vi "CRYGet Group Category.vi"(7 "sOption":string, 11 "nData":i32) -> (3 "sCategory":string)   [LabVIEW 2013]
uses:
  CRYProject/CRYProject Editor Global.vi
  Global/CRYCurve Library Global.vi
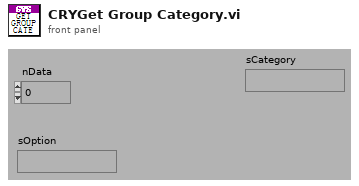
[diagram p1: front panel]
types:
  T1 = typedef "CRYStep.ctl" = cluster{"No.VI":i32, "Category":string, "StepName":string, "Seq setup flattened":string, "Comment":string, "Steps config.":bool[], "Jump config":i32[], "Start":dbl, "Increment":dbl, "Name":string, "Unit":string, "Y data":u16, "Y prefix":string, "Y dB ref":dbl, "Y unit":string, "Repeat State Array":cluster{"Start":dbl, "Increment":dbl, "Count":i32, "Num":i32}[]}
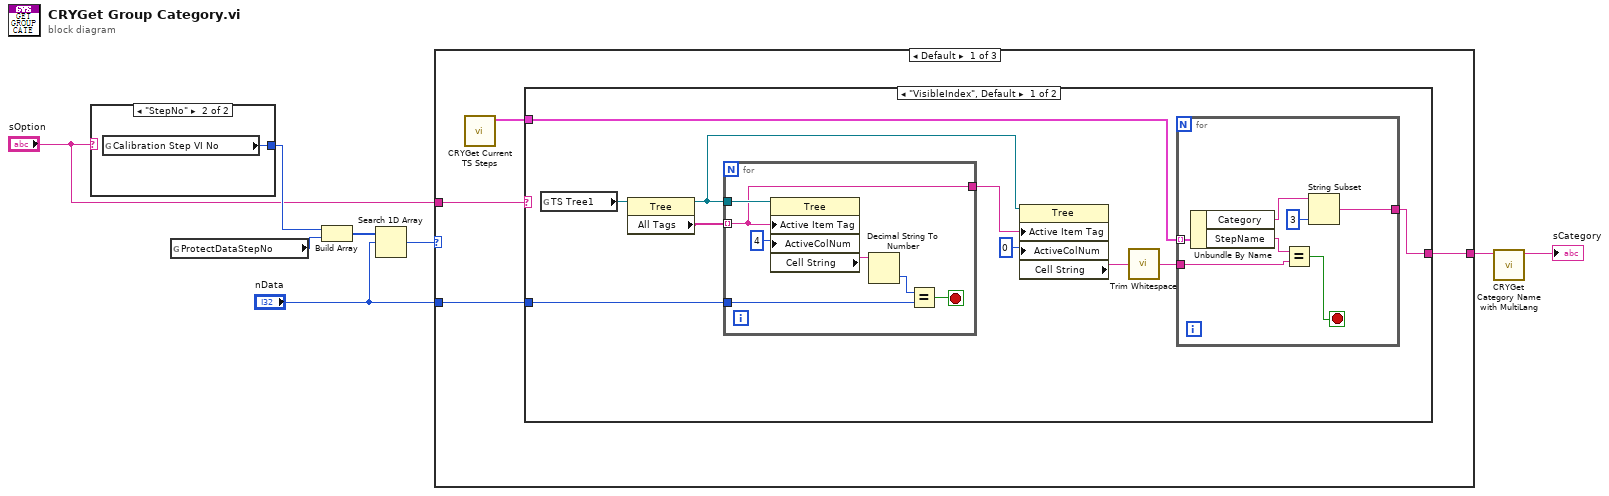
[diagram p0: block diagram]
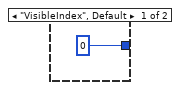
[diagram p2: hidden frame]
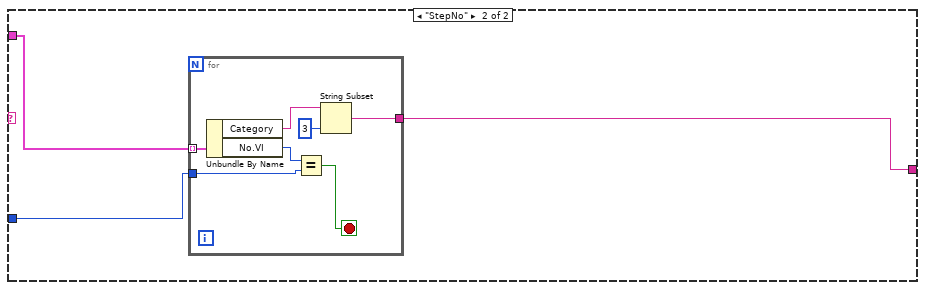
[diagram p3: hidden frame]
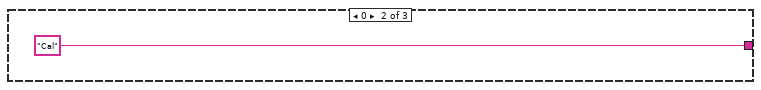
[diagram p4: hidden frame]
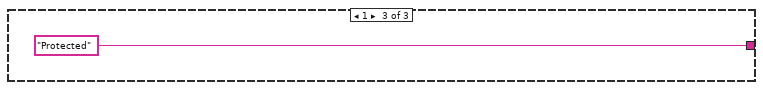
[diagram p5: hidden frame]
diagram:
  n1 = case shown="\"StepNo\"" "sOption" {
    tunnel: [0 ("element") w10] -> w4
    frame "VisibleIndex", Default {
    }
    frame "StepNo" {
      n2 = global read "CRYProject Editor Global.vi" "Calibration Step VI No"() -> (w10:i32)
    }
  }
  n3 = global read "CRYCurve Library Global.vi" "ProtectDataStepNo"() -> (w8:i32)
  n4 = Build Array(w4, w8) -> (w7:i32[])
  n5 = Search 1D Array(1D array=w7, element="nData") -> (index of element=w5:i32)  [unwired: 1 in]
  n6 = case shown="Default" w5 {
    tunnel: "nData" -> [w14 _ _]
    tunnel: [w12 "Cal" "Protected"] -> w2
    tunnel: "sOption" -> [w11 _ _]
    frame Default {
      n7 = call "CRYGet Current TS Steps.vi"() -> ("Steps"=w13:T1[])  [unwired: 7 in, 4 out]
      n8 = case shown="\"VisibleIndex\", Default" w11 {
        tunnel: w14 -> [w23 w39]
        tunnel: w13 -> [w22 w41]
        tunnel: [w21 w40] -> w12
        frame "VisibleIndex", Default {
          n9 = global read "CRYProject Editor Global.vi" "TS Tree1"() -> (w20:refnum<vi>)
          n10 = property class="Tree"(reference=w20) -> (reference out=w18:refnum<vi>, "All Tags"=w24:string[])  [unwired: 1 in, 1 out]
          n11 = for {
            tunnel: w24 -> [w32] mode=indexing
            tunnel: w23 -> [w35]
            tunnel: w18 -> [w38]
            tunnel: [w32] -> w19
            stop <- w34 stop-if-true
            n12 = property class="Tree"(reference=w38, "Active Item Tag"=w32, "ActiveColNum"=4 ("Active Cell:Active Column Number")) -> ("Cell String"=w37:string)  [unwired: 1 in, 2 out]
            n13 = Decimal String To Number(string=w37) -> (number=w36:i32)  [unwired: 2 in, 1 out]
            n14 = Equal?(x=w36, y=w35) -> (x = y?=w34:bool)
          }
          n15 = property class="Tree"(reference=w18, "Active Item Tag"=w19, "ActiveColNum"=0 ("Active Cell:Active Column Number")) -> ("Cell String"=w16:string)  [unwired: 1 in, 2 out]
          n16 = call <vilib>:"Trim Whitespace.vi"("string"=w16) -> ("trimmed string"=w15:string)  [unwired: 1 in]
          n17 = for {
            tunnel: w22 -> [w31] mode=indexing
            tunnel: w15 -> [w29]
            tunnel: [w25] -> w21
            stop <- w28 stop-if-true
            n18 = Unbundle By Name(w31) -> ("Category"=w26:string, "StepName"=w30:string)
            n19 = Equal?(x=w30, y=w29) -> (x = y?=w28:bool)
            n20 = String Subset(string=w26, length (rest)=3 ("length (rest)")) -> (substring=w25:string)  [unwired: 1 in]
          }
        }
        frame "StepNo" {
          n21 = for {
            tunnel: w41 -> [w48] mode=indexing
            tunnel: w39 -> [w46]
            tunnel: [w42] -> w40
            stop <- w45 stop-if-true
            n22 = Unbundle By Name(w48) -> ("Category"=w43:string, "No.VI"=w47:i32)
            n23 = Equal?(x=w47, y=w46) -> (x = y?=w45:bool)
            n24 = String Subset(string=w43, length (rest)=3 ("length (rest)")) -> (substring=w42:string)  [unwired: 1 in]
          }
        }
      }
    }
    frame 0 {
    }
    frame 1 {
    }
  }
  n25 = call "CRYGet Category Name with MultiLang.vi"("Category"=w2) -> ("Name"=→"sCategory":string)  [unwired: 10 in]
